vi "Grubbs_Test.vi"() -> ()   [LabVIEW 2013]
uses:
  Grubbs_Test_States.ctl
  <vilib>/Utility/file.llb/Read From Spreadsheet File (DBL).vi
  <vilib>/Analysis/NI_AALBase.lvlib
panel:
  out "Обработанные результаты":dbl[](graph)
  out "Исходная выборка":dbl[](graph)
  out "СКО":dbl
  out "Среднее":dbl
  out "Array":dbl[](array[numeric])
  in  "Уровень значимости":dbl
  in  "Путь к файлу данных":path
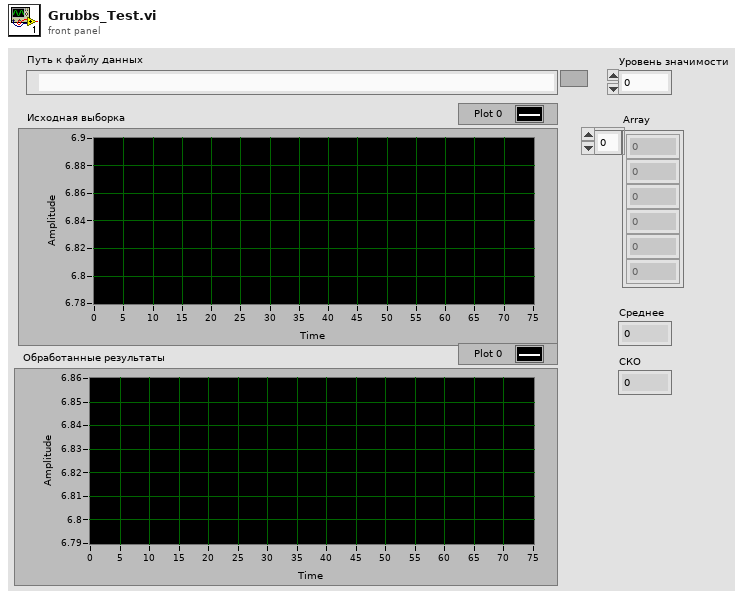
[diagram p1: front panel]
types:
  T1 = typedef "Grubbs_Test_States.ctl" = enum16{"Инициализация", "Расчет ошибок", "Проверка на промахи", "Завершение работы"}
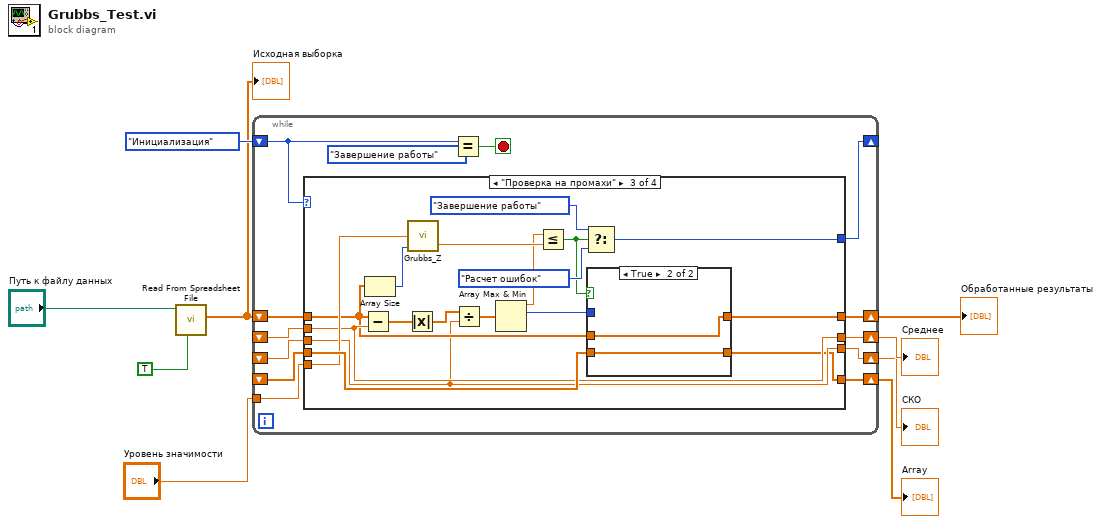
[diagram p0: block diagram]
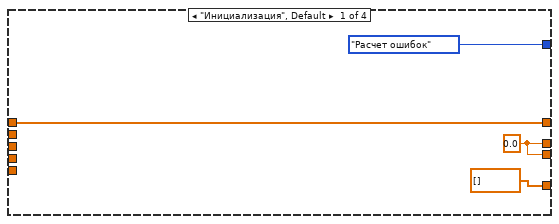
[diagram p2: hidden frame]
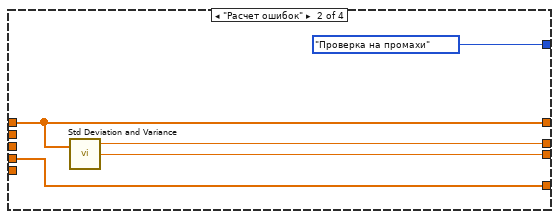
[diagram p3: hidden frame]
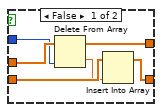
[diagram p4: hidden frame]
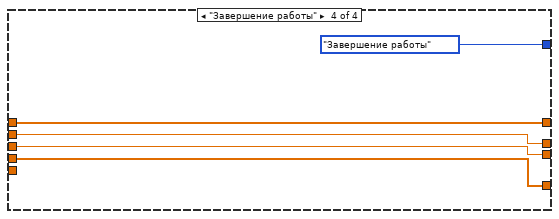
[diagram p5: hidden frame]
diagram:
  n1 = call-poly <vilib>:"Read From Spreadsheet File.vi"("transpose (no:F)"=TRUE, "file path (dialog if empty)"="Путь к файлу данных") -> ("first row"=w3:dbl[])  [unwired: 5 in, 4 out]
  "Исходная выборка" <- w3
  n2 = while {
    shift-right: [w22] -> _
    shift-left: Grubbs_Test_States."Инициализация" -> [w20]
    shift-right: [w15] -> w2
    shift-left: w3 -> [w16]
    shift-right: [w10] -> w8
    shift-left: _ -> [w12]
    shift-right: [w18] -> w7
    shift-left: _ -> [w11]
    shift-right: [w14] -> w1
    shift-left: _ -> [w13]
    tunnel: "Уровень значимости" -> [w17]
    stop <- w19 stop-if-true
    n3 = case shown="\"Проверка на промахи\"" w20 {
      tunnel: [Grubbs_Test_States."Расчет ошибок" Grubbs_Test_States."Проверка на промахи" w45 Grubbs_Test_States."Завершение работы"] -> w22
      tunnel: [w25 w28 w37 w60] -> w18
      tunnel: w17 -> [_ _ w41 _]
      tunnel: [w24 w30 w33 w62] -> w15
      tunnel: w16 -> [w24 w30 w38 w62]
      tunnel: [dbl[] [] w31 w32 w59] -> w14
      tunnel: w13 -> [_ w31 w49 w59]
      tunnel: w12 -> [_ _ w39 w61]
      tunnel: w11 -> [_ _ w37 w60]
      tunnel: [w25 w29 w39 w61] -> w10
      frame "Инициализация", Default {
        w25 = 0.0
      }
      frame "Расчет ошибок" {
        n4 = call <vilib>:"Std Deviation and Variance.vi"("X"=w30) -> ("mean"=w29:dbl, "standard deviation"=w28:dbl)  [unwired: 1 in, 1 out]
      }
      frame "Проверка на промахи" {
        n5 = Subtract(x=w38, y=w39) -> (x-y=w40:dbl[])
        n6 = Array Size(array=w38) -> (size(s)=w42:i32)
        n7 = Absolute Value(x=w40) -> (abs(x)=w48:dbl[])
        n8 = call "Grubbs_Z.vi"("n"=w42, "q"=w41) -> ("G"=w43:dbl)  [unwired: 2 in]
        n9 = Divide(x=w48, y=w37) -> (x/y=w36:dbl[])
        n10 = Array Max & Min(array=w36) -> (max value=w35:dbl, max index (indices)=w34:i32)  [unwired: 2 out]
        n11 = Less Or Equal?(x=w35, y=w43) -> (x <= y?=w44:bool)
        n12 = Select(t=Grubbs_Test_States."Завершение работы", s=w44, f=Grubbs_Test_States."Расчет ошибок") -> (s? t:f=w45:T1)
        n13 = case shown="True" w44 {
          tunnel: w38 -> [w55 w57]
          tunnel: [w54 w57] -> w33
          tunnel: w49 -> [w53 w56]
          tunnel: [w52 w56] -> w32
          tunnel: w34 -> [w50 _]
          frame False {
            n14 = Delete From Array(array=w55, index=w50) -> (deleted portion=w51:dbl, array with subset deleted=w54:dbl[])  [unwired: 1 in]
            n15 = Insert Into Array(array=w53, new element=w51) -> (w52:dbl[])  [unwired: 1 in]
          }
          frame True {
          }
        }
      }
      frame "Завершение работы" {
      }
    }
    n16 = Equal?(x=w20, y=Grubbs_Test_States."Завершение работы") -> (x = y?=w19:bool)
  }
  "Array" <- w1
  "Среднее" <- w8
  "СКО" <- w7
  "Обработанные результаты" <- w2
